vi "MEMORIA hp3458.vi"(4 "Distancia entre muestras (seg)":dbl format="%_4e", 8 "error in (no error)":errorcluster, 9 "Output Format (0:ASCII)":T1(ring)=enum."Single Integer", 10 "Número de muestras totales":dbl, 11 "VISA session":refnum<visa-resource-name>) -> (0 "error out":errorcluster, 1 "Muestras digitales":dbl[](array[numeric]) format="%^.3e", 2 "Array":cluster{dbl, "data":dbl}[](array[cluster]), 3 "dup VISA session":refnum<visa-resource-name>)   [LabVIEW 2014, in "SamplerPlugins.lvlib" / "HP3458aDMM.lvclass"]
uses:
  HP3458aDMM.lvclass
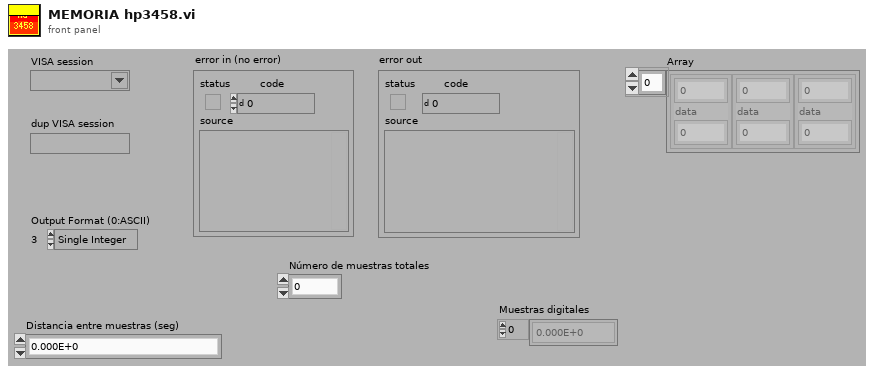
[diagram p1: front panel]
types:
  T1 = enum16{"ASCII", "Single Real", "Double Real", "Single Integer", "Double Integer"}
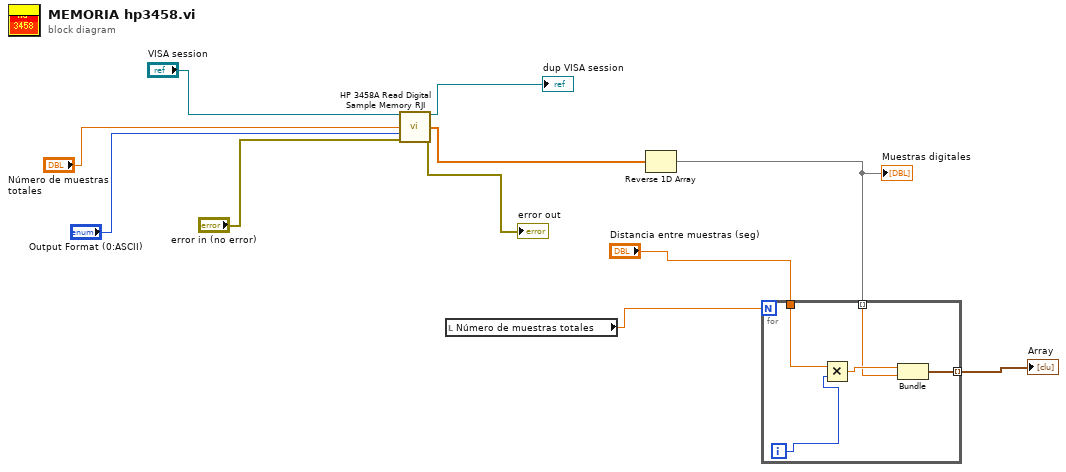
[diagram p0: block diagram]
diagram:
  n1 = call "HP 3458A Read Digital Sample Memory RJI.vi"("VISA session"="VISA session", "Numbers of Samples (100)"="Número de muestras totales", "Output Format (0:ASCII)"="Output Format (0:ASCII)", "error in (no error)"="error in (no error)") -> ("dup VISA session"=→"dup VISA session":refnum<visa-resource-name>, "Output Array"=w2:dbl[], "error out"=→"error out":errorcluster)  [unwired: 9 in]
  n2 = local read "Número de muestras totales"() -> (w9:dbl)
  n3 = Reverse 1D Array(array=w2) -> (reversed array=w8:dbl[])
  "Muestras digitales" <- w8
  n4 = for {
    N: w9 -> [_]
    tunnel: [w15] -> w11 mode=indexing
    tunnel: "Distancia entre muestras (seg)" -> [w13]
    tunnel: w8 -> [w12] mode=indexing
    i -> [w16]
    n5 = Multiply(x=w13, y=w16) -> (x*y=w14:dbl)
    n6 = Bundle(w14, "data"=w12) -> (w15:cluster{dbl, "data":dbl})  [unwired: 1 in]
  }
  "Array" <- w11
